vi "Main.vi"(11 "Module Admin":refnum<class "Delacor_lib_QMH_Module Admin.lvclass">) -> ()   [LabVIEW 2021, in "FunctionGenerator.lvlib"]
doc: "This template is based off of the Queued Message Handler design pattern and the Queued Message Handler project template that ships with LabVIEW.\n\nThe main difference is that the queue is private to this module and communication between modules is performed via Broadcast and Request events.\n\nRequest events are wrapped in public API methods and are handled in the Event Handling Loop (EHL) of this VI. Any module can register for Broadcast events sent by this module. The EHL generates messages based on user interface actions.\n\nThe Message Handling Loop (MHL) processes messages generated by the EHL, or by other messages. The messages are string values, so new messages can be added easily to the Message Cases case structure in the MHL. Each message cluster can also provide an optional value for Message Data, which is a variant that can be converted to whatever message-specific data is required.\n_____\nBased on DQMH Project Template 6.1.0.94."
uses:
  FunctionGenerator.lvlib
  <vilib>/Delacor/Delacor QMH/Libraries/Module Admin_class/Delacor_lib_QMH_Module Admin.lvclass
  Module Data--cluster.ctl
  <vilib>/Delacor/Delacor QMH/Libraries/Message Queue_class/Delacor_lib_QMH_Message Queue.lvclass/Delacor_lib_QMH_Message Queue.ctl
  Stop Argument--cluster.ctl
  <vilib>/Delacor/Delacor QMH/Libraries/Module Admin_class/Delacor_lib_QMH_Module Admin.lvclass/Delacor_lib_QMH_Module Admin.ctl
  Set Signal Type Argument--cluster.ctl
  Get Waveform Argument--cluster.ctl
  Get Waveform (Reply Payload)--cluster.ctl
  Set Frecuency Argument--cluster.ctl
  Offset Argument--cluster.ctl
  Amplitud Argument--cluster.ctl
  <vilib>/Utility/miscctls.llb/LVPointTypeDef.ctl
  <vilib>/Delacor/Delacor QMH/Libraries/Message Queue_class/Delacor_lib_QMH_Enqueue Message (Single).vi
  <vilib>/Delacor/Delacor QMH/Libraries/Module Admin_class/Delacor_lib_QMH_Get External Launch.vi
  <vilib>/Utility/error.llb/Error Cluster From Error Code.vi
  <vilib>/ErrorRing/Error Ring.xnode
  <vilib>/Delacor/Delacor QMH/Libraries/Message Queue_class/Delacor_lib_QMH_Message Queue.lvclass
  <vilib>/measure/NI_MABase.lvlib
panel:
  out "error out":errorcluster
  out "Status":string
  in  "Simulate MHL Error":bool
  in  "Simulate EHL Error":bool
  # "Other QMH Modules communicate with this Module via its Public API (wrappers for its Request Events).\n\nThis Module communicates with other Modules via its Broadcast Events.\nAny module that wants to get these messages, just registers for this module's Broadcast events."
  # "This template is for the Delacor Modified Queued Message Handler design pattern.\n\nSee the block diagram for more information on how to use this template."
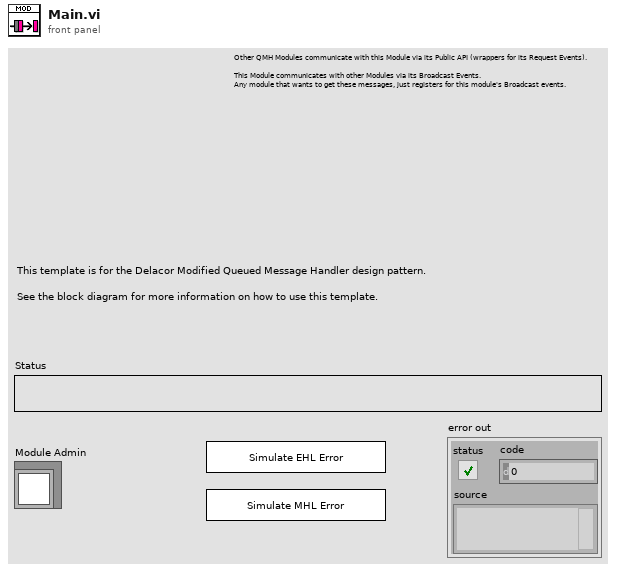
[diagram p1: front panel]
types:
  T1 = typedef "FunctionGenerator.lvlib/Request Events--cluster.ctl" = cluster{"Stop Module":refnum<user-event>, "Show Panel":refnum<user-event>, "Hide Panel":refnum<user-event>, "Get Module Execution Status":refnum<user-event>, "Show Diagram":refnum<user-event>, "Set Signal Type":refnum<user-event>, "Get Waveform":refnum<user-event>, "Set Frecuency":refnum<user-event>, "Offset":refnum<user-event>, "Amplitud":refnum<user-event>}
  T2 = typedef "FunctionGenerator.lvlib/Module Data--cluster.ctl" = cluster{"Status":string, "signal type":enum16{"Sine Wave", "Triangle Wave", "Square Wave", "Sawtooth Wave"}, "Frecuency":dbl, "Offset":dbl, "Amplitude":dbl}
  T3 = enum32{"invalid lock state", "Not Locked", "Locked (No Password)", "Password-protected"}
  T4 = typedef "FunctionGenerator.lvlib/Stop Argument--cluster.ctl" = cluster{"Origin":string, "Exit via Stop Module Req?":bool, "Wait for Module to stop?":bool}
  T5 = typedef "FunctionGenerator.lvlib/Set Signal Type Argument--cluster.ctl" = cluster{"signal type":enum16{"Sine Wave", "Triangle Wave", "Square Wave", "Sawtooth Wave"}}
  T6 = typedef "FunctionGenerator.lvlib/Get Waveform Argument--cluster.ctl" = cluster{"Wait Notifier":refnum<notifier>, "wait for reply":bool}
  T7 = typedef "FunctionGenerator.lvlib/Set Frecuency Argument--cluster.ctl" = cluster{"Frecuency":dbl}
  T8 = typedef "FunctionGenerator.lvlib/Offset Argument--cluster.ctl" = cluster{"Offset":dbl}
  T9 = typedef "FunctionGenerator.lvlib/Amplitud Argument--cluster.ctl" = cluster{"Amplitude":dbl}
  T10 = typedef "LVPointTypeDef.ctl" = cluster{"Horizontal":i16, "Vertical":i16}
  T11 = enum32{"Invalid", "Standard", "Closed", "Hidden", "Minimized", "Maximized"}
  T12 = typedef "FunctionGenerator.lvlib/Get Waveform (Reply Payload)--cluster.ctl" = cluster{"signal out":waveform(dbl), "error":errorcluster}
  T13 = enum16{"Sine Wave", "Triangle Wave", "Square Wave", "Sawtooth Wave"}
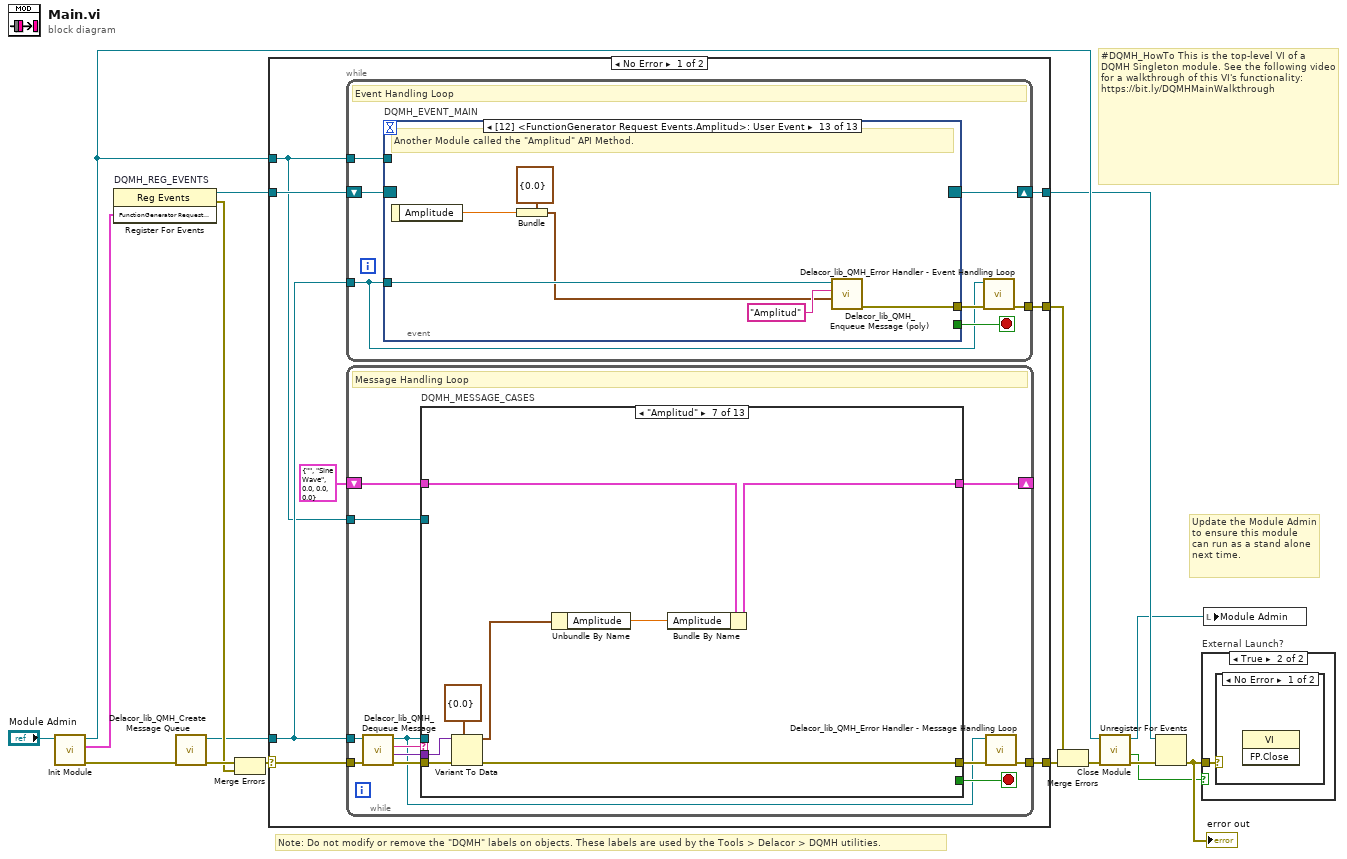
[diagram p0: block diagram]
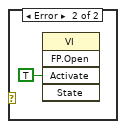
[diagram p3: hidden frame]
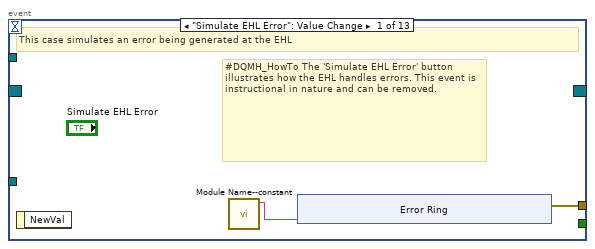
[diagram p4: hidden frame]
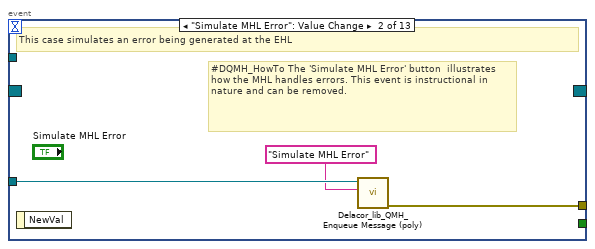
[diagram p5: hidden frame]
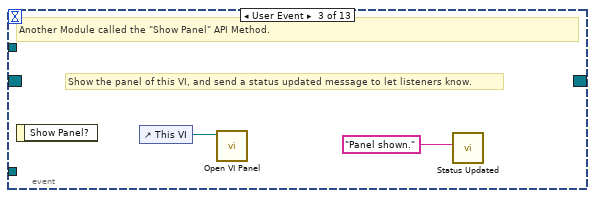
[diagram p6: hidden frame]
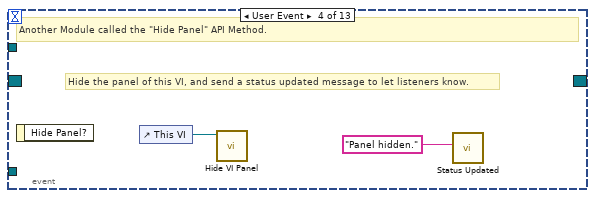
[diagram p7: hidden frame]
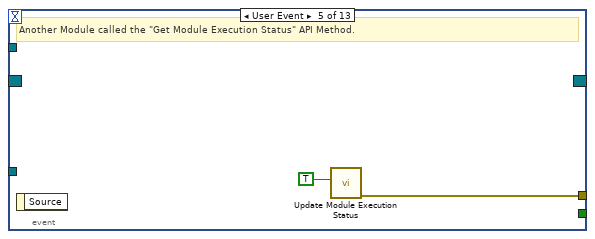
[diagram p8: hidden frame]
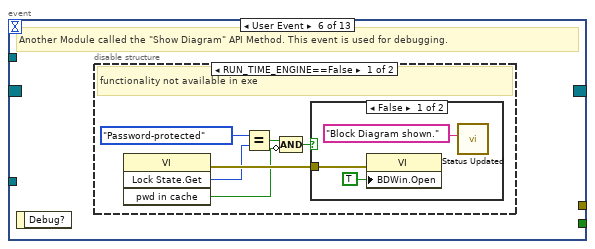
[diagram p9: hidden frame]
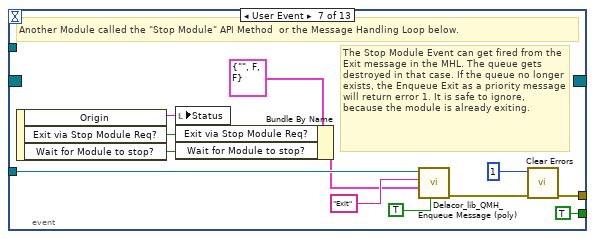
[diagram p12: hidden frame]
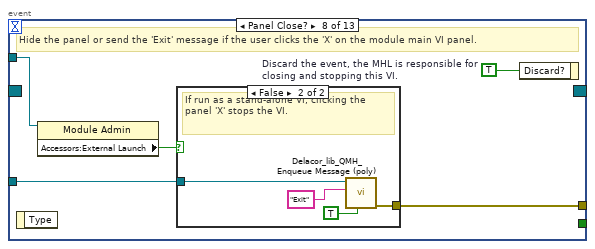
[diagram p13: hidden frame]
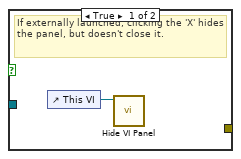
[diagram p14: hidden frame]
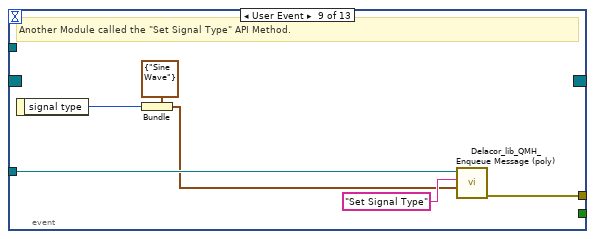
[diagram p15: hidden frame]
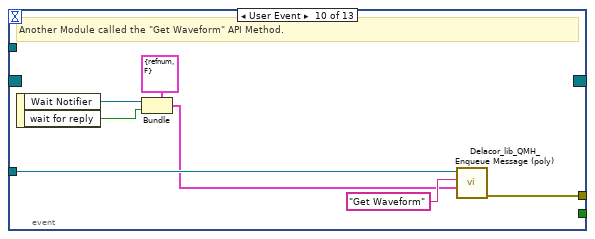
[diagram p16: hidden frame]
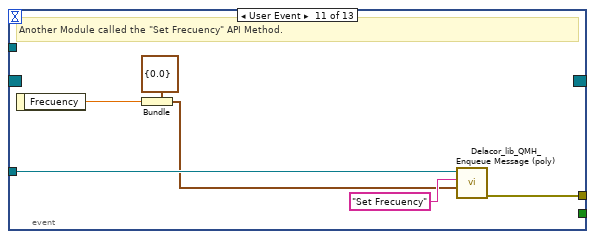
[diagram p17: hidden frame]
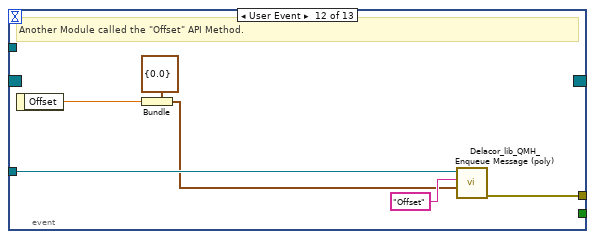
[diagram p18: hidden frame]
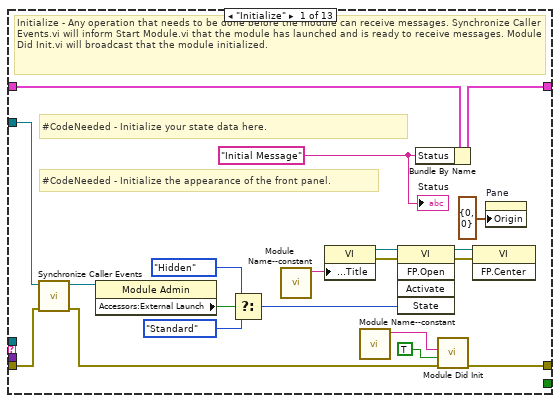
[diagram p19: hidden frame]
diagram:
  # "#DQMH_HowTo This is the top-level VI of a DQMH Singleton module. See the following video for a walkthrough of this VI's functionality: https://bit.ly/DQMHMainWalkthrough"
  # "Note: Do not modify or remove the \"DQMH\" labels on objects. These labels are used by the Tools > Delacor > DQMH utilities."
  # "Update the Module Admin to ensure this module can run as a stand alone next time."
  n1 = call "Init Module.vi"("Singleton Module Admin in"="Module Admin") -> ("error out"=w16:errorcluster, "FunctionGenerator Request Events"=w5:T1, "Singleton Module Admin out"=w8:refnum<class "Delacor_lib_QMH_Module Admin.lvclass">)  [unwired: 8 in]
  n2 = register-events "DQMH_REG_EVENTS"(w5) -> (reference out=w6:refnum<event-registration>, error out=w9:errorcluster)  [unwired: 2 in]
  n3 = call <vilib>:"Delacor_lib_QMH_Create Message Queue.vi"("error in"=w16) -> ("error out"=w11:errorcluster, "Message Queue"=w4:refnum<class "Delacor_lib_QMH_Message Queue.lvclass">)  [unwired: 9 in]
  n4 = Merge Errors(w11, w9) -> (w10:errorcluster)
  n5 = case shown="No Error" w10 {
    selector: w10 -> [w23 w259]
    tunnel: [w25 w258] -> w17
    tunnel: [w22 w264] -> w7
    tunnel: w6 -> [w20 w264]
    tunnel: w4 -> [w19 w257]
    tunnel: [w24 _] -> w14
    tunnel: w8 -> [w18 w260]
    frame No Error {
      n6 = while {
        tunnel: w19 -> [w26]
        shift-right: [w29] -> w22
        shift-left: w20 -> [w30]
        tunnel: [w31] -> w24
        tunnel: w18 -> [w27]
        stop <- w28 stop-if-true
        # "Event Handling Loop"
        n7 = event "DQMH_EVENT_MAIN" shown="[12] <FunctionGenerator Request Events.Amplitud>: User Event" {
          selector: w30 -> [_ _ _ _ _ _ _ _ _ _ _ _ _]
          dyn-events: [_ _ _ _ _ _ _ _ _ _ _ _ _] -> w29
          timeout: _ -> [_ _ _ _ _ _ _ _ _ _ _ _ _]
          tunnel: [_ _ _ _ _ _ TRUE ("Discard?") _ _ _ _ _ _] -> w28
          tunnel: w26 -> [_ w43 _ _ _ _ w67 w74 w87 w94 w100 w106 w112]
          tunnel: [w34 w44 _ _ w50 _ w70 w76 w82 w88 w95 w101 w107] -> w32
          tunnel: w27 -> [_ _ _ _ _ _ _ w73 _ _ _ _ _]
          event "Simulate EHL Error": Value Change {
            # "#DQMH_HowTo The 'Simulate EHL Error' button  illustrates how the EHL handles errors. This event is instructional in nature and can be removed."
            # "This case simulates an error being generated at the EHL"
            n8 = event-data() -> ()  [unwired: 1 in, 1 out]
            n9 = call "Module Name--constant.vi"() -> ("Module Name"=w33:string)  [unwired: 11 in]
            n10 = xnode "Error Ring"("parameter 0"=w33) -> ("error out"=w34:errorcluster)
          }
          event "Simulate MHL Error": Value Change {
            # "#DQMH_HowTo The 'Simulate MHL Error' button  illustrates how the MHL handles errors. This event is instructional in nature and can be removed."
            # "This case simulates an error being generated at the EHL"
            n11 = event-data() -> ()  [unwired: 1 in, 1 out]
            n12 = call-poly <vilib>:"Delacor_lib_QMH_Enqueue Message (poly).vi"("Message"="Simulate MHL Error", "Message Queue in"=w43) -> ("error out"=w44:errorcluster)  [unwired: 8 in, 1 out]
          }
          event User Event {
            # "Show the panel of this VI, and send a status updated message to let listeners know."
            # "Another Module called the \"Show Panel\" API Method."
            n13 = event-data() -> ()  [unwired: 1 in, 1 out]
            n14 = control-ref of="This VI"() -> (w46:refnum<vi>)
            n15 = call "Open VI Panel.vi"("VI"=w46) -> ()  [unwired: 10 in, 1 out]
            n16 = call "Status Updated.vi"("Status"="Panel shown." ("format string")) -> ()  [unwired: 10 in, 1 out]
          }
          event User Event {
            # "Hide the panel of this VI, and send a status updated message to let listeners know."
            # "Another Module called the \"Hide Panel\" API Method."
            n17 = event-data() -> ()  [unwired: 1 in, 1 out]
            n18 = control-ref of="This VI"() -> (w48:refnum<vi>)
            n19 = call "Hide VI Panel.vi"("VI"=w48) -> ()  [unwired: 10 in, 1 out]
            n20 = call "Status Updated.vi"("Status"="Panel hidden." ("format string")) -> ()  [unwired: 10 in, 1 out]
          }
          event User Event {
            # "Another Module called the \"Get Module Execution Status\" API Method."
            n21 = event-data() -> ()  [unwired: 1 in, 1 out]
            n22 = call "Update Module Execution Status.vi"("Running?"=TRUE) -> ("error out"=w50:errorcluster)  [unwired: 10 in]
          }
          event User Event {
            # "Another Module called the \"Show Diagram\" API Method. This event is used for debugging."
            n23 = event-data() -> ()  [unwired: 1 in, 1 out]
            n24 = disable-structure shown="RUN_TIME_ENGINE==False" {
              frame condition #0 (active) {
                # "functionality not available in exe"
                n25 = invoke class="VI" method="Lock State.Get"() -> (error out=w56:errorcluster, "Get Lock State"=w55:T3, "pwd in cache"=w52:bool)  [unwired: 4 in, 1 out]
                n26 = Equal?(x=T3."Password-protected", y=w55) -> (x = y?=w53:bool)
                n27 = Compound Arithmetic op=AND(w53, invert w52) -> (w51:bool)
                n28 = case shown="False" w51 {
                  tunnel: w56 -> [w59 _]
                  frame False {
                    n29 = property class="VI"(error in=w59, "BDWin.Open"=TRUE ("Block Diagram Window:Open")) -> ()  [unwired: 1 in, 2 out]
                    n30 = call "Status Updated.vi"("Status"="Block Diagram shown." ("format string")) -> ()  [unwired: 10 in, 1 out]
                  }
                  frame True {
                    # "Password-protected VI, and the password is not in the cache. Do not show the diagram."
                  }
                }
              }
              frame condition #1 {
              }
            }
          }
          event User Event {
            # "The Stop Module Event can get fired from the Exit message in the MHL. The queue gets destroyed in that case. If the queue no longer exists, the Enqueue Exit as a priority message will return error 1. It is safe to ignore, because the module is already exiting."
            # "Another Module called the \"Stop Module\" API Method  or the Message Handling Loop below."
            n31 = event-data() -> ("Origin"=w66:string, "Exit via Stop Module Req?"=w62:bool, "Wait for Module to stop?"=w61:bool)  [unwired: 1 in]
            n32 = local write "Status"(w66) -> ()
            n33 = Bundle By Name(cluster=T4 {"Origin"="", "Exit via Stop Module Req?"=FALSE, "Wait for Module to stop?"=FALSE} ("Stop Argument"), "Exit via Stop Module Req?"=w62, "Wait for Module to stop?"=w61) -> (w60:T4)
            n34 = call-poly <vilib>:"Delacor_lib_QMH_Enqueue Message (poly).vi"("Priority Message? (F)"=TRUE, "Message Data"=w60, "Message"="Exit", "Message Queue in"=w67) -> ("error out"=w71:errorcluster)  [unwired: 6 in, 1 out]
            n35 = call <vilib>:"Clear Errors.vi"("error in (no error)"=w71, "specific error code to clear (0: all)"=1) -> ("error out"=w70:errorcluster)  [unwired: 4 in, 1 out]
          }
          event Panel Close? {
            w75 = TRUE  # Discard the event, the MHL is responsible for closing and stopping this VI.
            # "Hide the panel or send the 'Exit' message if the user clicks the 'X' on the module main VI panel."
            n36 = event-data() -> ()  [unwired: 1 in, 1 out]
            n37 = property class="Module Admin"(reference=w73) -> ("Accessors:External Launch"=w72:bool)  [unwired: 1 in, 2 out]
            n38 = case shown="False" w72 {
              tunnel: w74 -> [_ w80]
              tunnel: [_ w81] -> w76
              frame True {
                # "If externally launched, clicking the 'X' hides the panel, but doesn't close it."
                n39 = control-ref of="This VI"() -> (w77:refnum<vi>)
                n40 = call "Hide VI Panel.vi"("VI"=w77) -> ()  [unwired: 10 in, 1 out]
              }
              frame False {
                # "If run as a stand-alone VI, clicking the panel 'X' stops the VI."
                n41 = call-poly <vilib>:"Delacor_lib_QMH_Enqueue Message (poly).vi"("Priority Message? (F)"=TRUE, "Message"="Exit", "Message Queue in"=w80) -> ("error out"=w81:errorcluster)  [unwired: 7 in, 1 out]
              }
            }
            n42 = event-data("Discard?"=w75) -> ()  [unwired: 1 in, 1 out]
          }
          event User Event {
            # "Another Module called the \"Set Signal Type\" API Method."
            n43 = event-data() -> ("signal type"=w83:T13)  [unwired: 1 in]
            n44 = Bundle(cluster=T5 {"signal type"=enum."Sine Wave"} ("Set Signal Type Argument"), "signal type"=w83) -> (w84:T5)
            n45 = call-poly <vilib>:"Delacor_lib_QMH_Enqueue Message (poly).vi"("Message Data"=w84, "Message"="Set Signal Type", "Message Queue in"=w87) -> ("error out"=w82:errorcluster)  [unwired: 7 in, 1 out]
          }
          event User Event {
            # "Another Module called the \"Get Waveform\" API Method."
            n46 = event-data() -> ("Wait Notifier"=w90:refnum<notifier>, "wait for reply"=w89:bool)  [unwired: 1 in]
            n47 = Bundle(cluster=T6 {"Wait Notifier"=refnum, "wait for reply"=FALSE} ("Get Waveform Argument"), "Wait Notifier"=w90, "wait for reply"=w89) -> (w91:T6)
            n48 = call-poly <vilib>:"Delacor_lib_QMH_Enqueue Message (poly).vi"("Message Data"=w91, "Message"="Get Waveform", "Message Queue in"=w94) -> ("error out"=w88:errorcluster)  [unwired: 7 in, 1 out]
          }
          event User Event {
            # "Another Module called the \"Set Frecuency\" API Method."
            n49 = event-data() -> ("Frecuency"=w96:dbl)  [unwired: 1 in]
            n50 = Bundle(cluster=T7 {"Frecuency"=0.0} ("Set Frecuency Argument"), "Frecuency"=w96) -> (w97:T7)
            n51 = call-poly <vilib>:"Delacor_lib_QMH_Enqueue Message (poly).vi"("Message Data"=w97, "Message"="Set Frecuency", "Message Queue in"=w100) -> ("error out"=w95:errorcluster)  [unwired: 7 in, 1 out]
          }
          event User Event {
            # "Another Module called the \"Offset\" API Method."
            n52 = event-data() -> ("Offset"=w102:dbl)  [unwired: 1 in]
            n53 = Bundle(cluster=T8 {"Offset"=0.0} ("Offset Argument"), "Offset"=w102) -> (w103:T8)
            n54 = call-poly <vilib>:"Delacor_lib_QMH_Enqueue Message (poly).vi"("Message Data"=w103, "Message"="Offset", "Message Queue in"=w106) -> ("error out"=w101:errorcluster)  [unwired: 7 in, 1 out]
          }
          event User Event {
            # "Another Module called the \"Amplitud\" API Method."
            n55 = event-data() -> ("Amplitude"=w108:dbl)  [unwired: 1 in]
            n56 = Bundle(cluster=T9 {"Amplitude"=0.0} ("Amplitud Argument"), "Amplitude"=w108) -> (w109:T9)
            n57 = call-poly <vilib>:"Delacor_lib_QMH_Enqueue Message (poly).vi"("Message Data"=w109, "Message"="Amplitud", "Message Queue in"=w112) -> ("error out"=w107:errorcluster)  [unwired: 7 in, 1 out]
          }
        }
        n58 = call-dynamic "Delacor_lib_QMH_Error Handler - Event Handling Loop.vi"("error in"=w32, "Message Queue in"=w26) -> ("dup error in"=w31:errorcluster)  [unwired: 8 in, 1 out]
      }
      n59 = while {
        tunnel: w19 -> [w115]
        shift-right: [w119] -> _
        shift-left: T2 {"Status"="", "signal type"=enum."Sine Wave", "Frecuency"=0.0, "Offset"=0.0, "Amplitude"=0.0} ("Data Cluster") -> [w120]
        tunnel: w23 -> [w123]
        tunnel: [w121] -> w25
        tunnel: w18 -> [w113]
        stop <- w118 stop-if-true
        # "Message Handling Loop"
        n60 = call-dynamic "Delacor_lib_QMH_Dequeue Message.vi"("error in"=w123, "Message Queue in"=w115) -> ("error out"=w122:errorcluster, "Message Data"=w116:variant, "Message"=w117:string, "Message Queue out"=w114:refnum<class "Delacor_lib_QMH_Message Queue.lvclass">)  [unwired: 6 in]
        n61 = case "DQMH_MESSAGE_CASES" shown="\"Amplitud\"" w117 {
          selector: w117 -> [_ _ _ _ _ _ _ _ _ _ _ _ w244]
          tunnel: w114 -> [_ _ _ _ _ _ _ _ _ _ w214 w236 _]
          tunnel: w122 -> [w142 w146 w154 w170 w178 w186 w194 w197 w199 w204 w221 w242 w246]
          tunnel: [w140 w146 w153 w161 w176 w184 w192 w196 w199 w203 w217 w239 w247] -> w124
          tunnel: w120 -> [w131 w145 w148 w160 w177 w185 w193 w195 w198 w201 w216 w235 w245]
          tunnel: [w130 w145 w147 w160 w177 w180 w188 w195 w198 w201 w216 w235 w245] -> w119
          tunnel: [_ _ _ _ _ _ _ _ _ _ _ w234 _] -> w118
          tunnel: w116 -> [_ _ w152 w168 w175 w183 w191 _ _ _ w215 w233 _]
          tunnel: w113 -> [w132 _ _ _ _ _ _ _ _ _ w213 w228 _]
          frame "Initialize" {
            w126 = "Initial Message" ("Initial Message")
            # "#CodeNeeded - Initialize the appearance of the front panel."
            # "#CodeNeeded - Initialize your state data here."
            # "Initialize - Any operation that needs to be done before the module can receive messages. Synchronize Caller Events.vi will inform Start Module.vi that the module has launched and is ready to receive messages. Module Did Init.vi will broadcast that the module initialized."
            n62 = call "Synchronize Caller Events.vi"("error in (no error)"=w142, "Singleton Module Admin in"=w132) -> ("error out"=w141:errorcluster, "Singleton Module Admin out"=w127:refnum<class "Delacor_lib_QMH_Module Admin.lvclass">)  [unwired: 8 in]
            n63 = property class="Module Admin"(reference=w127) -> ("Accessors:External Launch"=w136:bool)  [unwired: 1 in, 2 out]
            n64 = Select(t=T11."Hidden" ("State"), s=w136, f=T11."Standard" ("State")) -> (s? t:f=w133:T11)
            n65 = call "Module Name--constant.vi"() -> ("Module Name"=w139:string)  [unwired: 11 in]
            n66 = property class="VI"("Front Panel.Title"=w139) -> (reference out=w138:refnum<vi>, error out=w144:errorcluster)  [unwired: 2 in]
            n67 = call "Module Name--constant.vi"() -> ("Module Name"=w128:string)  [unwired: 11 in]
            n68 = invoke class="VI" method="FP.Open"(reference=w138, error in=w144, "State"=w133) -> (reference out=w137:refnum<vi>, error out=w143:errorcluster)  [unwired: 2 in, 3 out]
            n69 = Bundle By Name(cluster=w131, "Status"=w126) -> (w130:T2)
            n70 = call "Module Did Init.vi"("error in (no error)"=w141, "Initialized?"=TRUE, "Origin"=w128) -> ("error out"=w140:errorcluster)  [unwired: 8 in]
            n71 = invoke class="VI" method="FP.Center"(reference=w137, error in=w143) -> ()  [unwired: 1 in, 3 out]
            n72 = property on="Pane" class="Pane"("Origin"=T10 {"Horizontal"=0, "Vertical"=0}) -> ()  [unwired: 2 in, 2 out]
            "Status" <- w126
          }
          frame "---Module Specific---" {
            # "Separator -- The following cases handle messages specific to this Module."
          }
          frame "Set Signal Type" {
            # "Request al módulo para selección del tipo de función a generar."
            n73 = Variant To Data(error in=w154, type=T5 {"signal type"=enum."Sine Wave"} ("Set Signal Type Argument"), Variant=w152) -> (data=w150:T5, error out=w153:errorcluster)
            n74 = Unbundle By Name(w150) -> ("signal type"=w149:T13)
            n75 = Bundle By Name(cluster=w148, "signal type"=w149) -> (w147:T2)
          }
          frame "Get Waveform" {
            n76 = Variant To Data(error in=w170, type=T6 {"Wait Notifier"=refnum, "wait for reply"=FALSE} ("Get Waveform Argument"), Variant=w168) -> (data=w166:T6, error out=w169:errorcluster)
            n77 = Unbundle By Name(w160) -> ("Offset"=w157:dbl, "signal type"=w159:T13, "Frecuency"=w158:dbl)
            n78 = Unbundle By Name(w166) -> ("Wait Notifier"=w165:refnum<notifier>, "wait for reply"=w164:bool)
            n79 = call <vilib>:"Basic Function Generator.vi"("offset"=w157, "signal type"=w159, "frequency"=w158) -> ("error out"=w156:errorcluster, "signal out"=w155:waveform(dbl))  [unwired: 6 in, 1 out]
            n80 = call "New Waveform was acquired.vi"("error in"=w156, "signal out"=w155) -> ()  [unwired: 9 in, 1 out]
            n81 = Bundle By Name(cluster=T12 {"signal out"={"t0"=timestamp(0 s since 1904-01-01), "dt"=1.0, "Y"=[]}, "error"={"status"=FALSE, "code"=0, "source"=""}} ("Get Waveform (Reply Payload)"), "signal out"=w155, "error"=w156) -> (w163:T12)
            n82 = Merge Errors(w156, w169) -> (w161:errorcluster)
            n83 = case shown="True" w164 {
              tunnel: w165 -> [_ w172]
              tunnel: w163 -> [_ w171]
              frame False {
              }
              frame True {
                n84 = Send Notification(notification=w171, notifier=w172) -> ()  [unwired: 1 in, 2 out]
              }
            }
          }
          frame "Set Frecuency" {
            # "#CodeNeeded\n1. Configure this Message Case for handling the \"Set Frecuency\" message.\n2. Delete or edit this label when done."
            n85 = Variant To Data(error in=w178, type=T7 {"Frecuency"=0.0} ("Set Frecuency Argument"), Variant=w175) -> (data=w173:T7, error out=w176:errorcluster)
            n86 = Unbundle By Name(w173) -> ()  [unwired: 1 out]
          }
          frame "Offset" {
            n87 = Variant To Data(error in=w186, type=T8 {"Offset"=0.0} ("Offset Argument"), Variant=w183) -> (data=w181:T8, error out=w184:errorcluster)
            n88 = Unbundle By Name(w181) -> ("Offset"=w179:dbl)
            n89 = Bundle By Name(cluster=w185, "Frecuency"=w179) -> (w180:T2)
          }
          frame "Amplitud" {
            n90 = Variant To Data(error in=w194, type=T9 {"Amplitude"=0.0} ("Amplitud Argument"), Variant=w191) -> (data=w189:T9, error out=w192:errorcluster)
            n91 = Unbundle By Name(w189) -> ("Amplitude"=w187:dbl)
            n92 = Bundle By Name(cluster=w193, "Amplitude"=w187) -> (w188:T2)
          }
          frame "---Copy This Frame---" {
            # "Duplicate this frame when creating new messages.  Change this comment in the duplicated frame to describe this message."
            n93 = Merge Errors(w197) -> (w196:errorcluster)
          }
          frame "---Exit and Error Handling---" {
            # "Separator - The following cases handle errors and exit messages."
          }
          frame "Simulate MHL Error" {
            # "#DQMH_HowTo The 'Simulate MHL Error' button  illustrates how the MHL handles errors. This event is instructional in nature and can be removed."
            # "Simulate an error occurring at the MHL"
            n94 = call "Module Name--constant.vi"() -> ("Module Name"=w200:string)  [unwired: 11 in]
            n95 = xnode "Error Ring"("parameter 0"=w200) -> ("error out"=w202:errorcluster)
            n96 = Merge Errors(w204, w202) -> (w203:errorcluster)
          }
          frame "Error" {
            # "#CodeRecommended - If you ever change the name of this \"Error\" message, you'll need to update the name in the Check Loop Error.vi as well."
            # "#CodeRecommended - If the module is running in standalone mode (External Launch = FALSE), this code will pop up an error dialog and call the 'Exit' message if an error occurs. Add more fine-grained error handling here."
            # "Error - Check the error message data and respond accordingly. This message is sent by the \"Error Handler\" VIs at the end of each loop in this application."
            n97 = property class="Module Admin"(reference=w213) -> ("Accessors:External Launch"=w212:bool)  [unwired: 1 in, 2 out]
            n98 = Variant To Data(error in=w221, type=errorcluster {"status"=FALSE, "code"=0, "source"=""} ("error constant"), Variant=w215) -> (data=w222:errorcluster, error out=w219:errorcluster)
            n99 = call "Error Reported.vi"("Error"=w222) -> ()  [unwired: 10 in, 1 out]
            n100 = case shown="False" w212 {
              tunnel: [w227 _] -> w218
              tunnel: w214 -> [w225 _]
              tunnel: w222 -> [w226 _]
              frame False {
                # "If the module is running standalone, then pop up an error dialog and call the \"Exit\" message."
                n101 = call <vilib>:"Simple Error Handler.vi"("error in (no error)"=w226) -> ()  [unwired: 4 in, 5 out]
                n102 = call-poly <vilib>:"Delacor_lib_QMH_Enqueue Message (poly).vi"("Priority Message? (F)"=TRUE, "Message"="Exit", "Message Queue in"=w225) -> ("error out"=w227:errorcluster)  [unwired: 7 in, 1 out]
              }
              frame True {
                # "If the module was launched externally, calling the Error Reported broadcast VI is the only action performed by the \"Error\" message. The module's caller can then process the error appropriately."
              }
            }
            n103 = Merge Errors(w219, w218) -> (w217:errorcluster)
            n104 = local write "error out"(w217) -> ()
          }
          frame "Exit" {
            w232 = 91  # 91: not all Exit messages will have an argument
            w234 = TRUE  # Stop the VI
            # "Release the message queue reference"
            # "#CodeNeeded - Add any required cleanup code here"
            # "Exit - Exit the application."
            n105 = Variant To Data(error in=w242, type=T4 {"Origin"="", "Exit via Stop Module Req?"=FALSE, "Wait for Module to stop?"=FALSE} ("Stop Argument"), Variant=w233) -> (data=w230:T4, error out=w238:errorcluster)
            n106 = call <vilib>:"Clear Errors.vi"("error in (no error)"=w238, "specific error code to clear (0: all)"=w232) -> ("error out"=w241:errorcluster)  [unwired: 4 in, 1 out]
            n107 = control-ref of="This VI"() -> (w229:refnum<vi>)
            n108 = call-dynamic "Delacor_lib_QMH_Release Message Queue.vi"("error in"=w241, "Message Queue"=w236) -> ("error out"=w240:errorcluster)  [unwired: 9 in]
            n109 = call "Handle Exit.vi"("Stop Argument"=w230, "Admin in"=w228, "VI reference"=w229) -> ("error out"=w237:errorcluster)  [unwired: 7 in, 1 out]
            n110 = Merge Errors(w240, w237) -> (w239:errorcluster)
          }
          frame Default {
            # "'Default' case only runs if there is a message that isn't defined in any of the other cases.  Output a programming error."
            n111 = call "Module Name--constant.vi"() -> ("Module Name"=w243:string)  [unwired: 11 in]
            n112 = xnode "Error Ring"("parameter 0"=w244, "parameter 1"=w243) -> ("error out"=w248:errorcluster)
            n113 = Merge Errors(w246, w248) -> (w247:errorcluster)
          }
        }
        n114 = call-dynamic "Delacor_lib_QMH_Error Handler - Message Handling Loop.vi"("error in"=w124, "Message Queue in"=w114) -> ("dup error in"=w121:errorcluster)  [unwired: 8 in, 1 out]
      }
    }
    frame Error {
      # "Synchronize Caller Events.vi will inform Start Module.vi that the module has launched and will let the code calling Start Module.vi register for broadcasts and would permit the caller receive the broadcast that an error occurred at launch time."
      n115 = call-dynamic "Delacor_lib_QMH_Release Message Queue.vi"("error in"=w259, "Message Queue"=w257) -> ("error out"=w258:errorcluster)  [unwired: 9 in]
      n116 = call "Synchronize Caller Events.vi"("Singleton Module Admin in"=w260) -> ("error out"=w265:errorcluster)  [unwired: 9 in, 1 out]
      n117 = call "Module Name--constant.vi"() -> ("Module Name"=w263:string)  [unwired: 11 in]
      n118 = Format Into String(format string="An error occurred during initialization. %s is no longer running.", w263) -> (resulting string=w261:string)  [unwired: 2 in, 1 out]
      n119 = Merge Errors(w258, w265) -> (w266:errorcluster)
      n120 = call "Error Reported.vi"("Additional Information"=w261, "Error"=w266) -> ()  [unwired: 9 in, 1 out]
    }
  }
  n121 = Merge Errors(w14, w17) -> (w13:errorcluster)
  n122 = call "Close Module.vi"("error in (no error)"=w13, "Module Admin in"=w8) -> ("error out"=w15:errorcluster, "External Launch"=w1:bool, "Module Admin out"=w2:refnum<class "Delacor_lib_QMH_Module Admin.lvclass">)  [unwired: 7 in]
  n123 = Unregister For Events(event registration refnum=w7, error in=w15) -> (error out=w12:errorcluster)
  "error out" <- w12
  n124 = case "External Launch?" shown="True" w1 {
    tunnel: w12 -> [_ w267]
    frame False {
    }
    frame True {
      n125 = case shown="No Error" w267 {
        frame No Error {
          n126 = invoke class="VI" method="FP.Close"() -> ()  [unwired: 3 in, 3 out]
        }
        frame Error {
          n127 = invoke class="VI" method="FP.Open"("Activate"=TRUE ("Activate?")) -> ()  [unwired: 4 in, 5 out]
        }
      }
    }
  }
  n128 = local write "Module Admin"(w2) -> ()
